vi "Get Equation Para.vi"(8 "error in (no error)":errorcluster, 11 "PDE_2ndOrder_ConstPara in":refnum<class "NI_PDE_2ndOrder_ConstPara.lvclass">) -> (0 "error out":errorcluster, 2 "parameter":variant, 3 "PDE_2ndOrder_ConstPara out":refnum<class "NI_PDE_2ndOrder_ConstPara.lvclass">)   [LabVIEW 2020, in "NI_PDE.lvlib" / "NI_PDE_2ndOrder_ConstPara.lvclass"]
uses:
  <vilib>/gmath/pde.llb/PDEClass/PDE_2ndOrder_ConstPara/NI_PDE_2ndOrder_ConstPara.lvclass
  <vilib>/gmath/pde.llb/PDEClass/PDE_2ndOrder_ConstPara/Para Data.ctl
  <vilib>/gmath/pde.llb/PDEClass/PDE_2ndOrder_ConstPara/NI_PDE_2ndOrder_ConstPara.lvclass/NI_PDE_2ndOrder_ConstPara.ctl
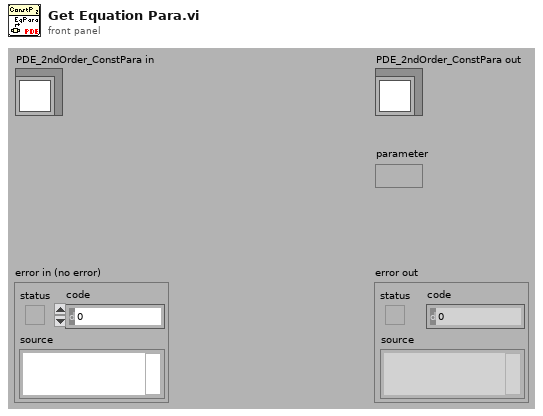
[diagram p1: front panel]
types:
  T1 = typedef "NI_PDE.lvlib/NI_PDE_2ndOrder_ConstPara.lvclass/Para Data.ctl" = cluster{"k":dbl, "a":dbl}
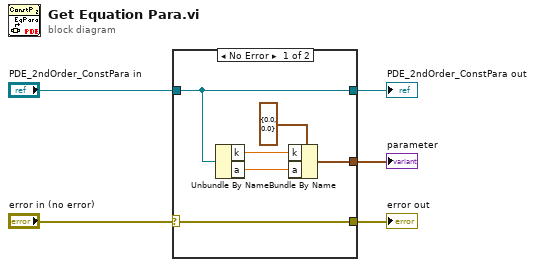
[diagram p0: block diagram]
diagram:
  n1 = case shown="No Error" "error in (no error)" {
    selector: "error in (no error)" -> [w6 w13]
    tunnel: "PDE_2ndOrder_ConstPara in" -> [w9 w12]
    tunnel: [w9 w12] -> w4
    tunnel: [w6 w13] -> w3
    tunnel: [w10 _] -> w1
    frame No Error {
      n2 = Unbundle By Name(w9) -> ("k"=w8:dbl, "a"=w7:dbl)
      n3 = Bundle By Name(cluster=T1 {"k"=0.0, "a"=0.0} ("para data"), "k"=w8, "a"=w7) -> (w10:T1)
    }
    frame Error {
    }
  }
  "PDE_2ndOrder_ConstPara out" <- w4
  "error out" <- w3
  "parameter" <- w1
